vi "new.vi"() -> ()   [LabVIEW 2019]
uses:
  <vilib>/Instr/_visa.llb/VISA Configure Serial Port (Instr).vi
panel:
  out "3.3V REG":cluster{dbl, dbl}(graph)
  out "3.3 current":dbl caption="Current Temperature\n(Celsius)"
  out "3.3V voltage":dbl caption="Current Temperature\n(Celsius)"
  out "5V REG":cluster{dbl, dbl}(graph)
  out "5V current":dbl caption="Current Temperature\n(Celsius)"
  out "Currents":cluster{dbl, dbl}(graph)
  in  "project name":string
  out "Bus Voltage":dbl(graph)
  out "5V voltage":dbl caption="Current Temperature\n(Celsius)"
  in  "StartConverter":bool
  out "String":string
  in  "VISA resource name":refnum<visa-resource-name>="COM4"
  out "LOAD current":dbl caption="Current Temperature\n(Celsius)"
  out "PVA current":dbl caption="Current Temperature\n(Celsius)"
  out "BUS voltage":dbl caption="Current Temperature\n(Celsius)"
  out "Still in Sync":bool
  in  "stop":bool
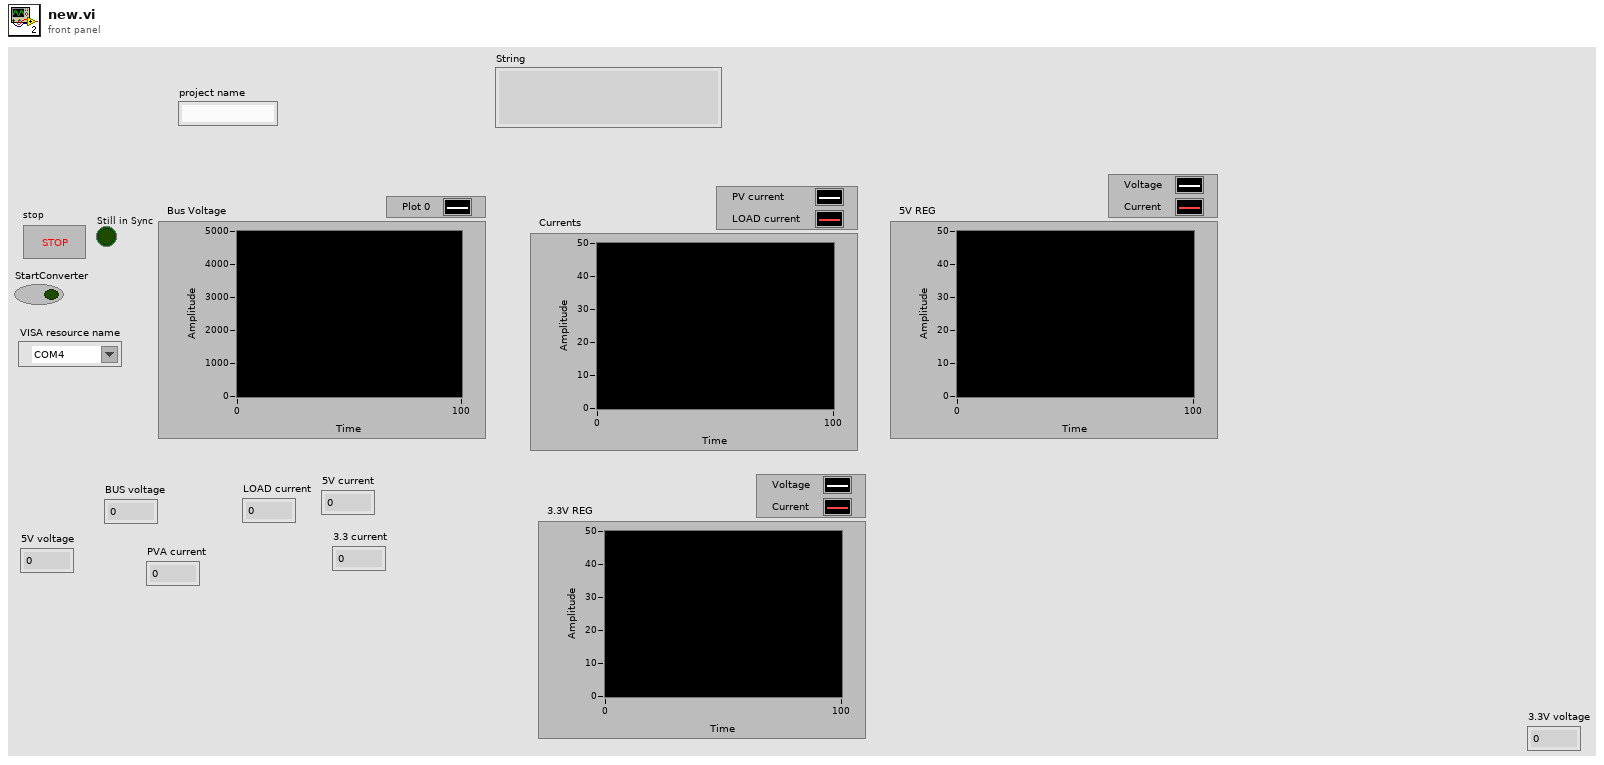
[diagram p1: front panel]
types:
  T1 = cluster{u16, u16, u16, u16, u16, u16, u16, u16, u16}
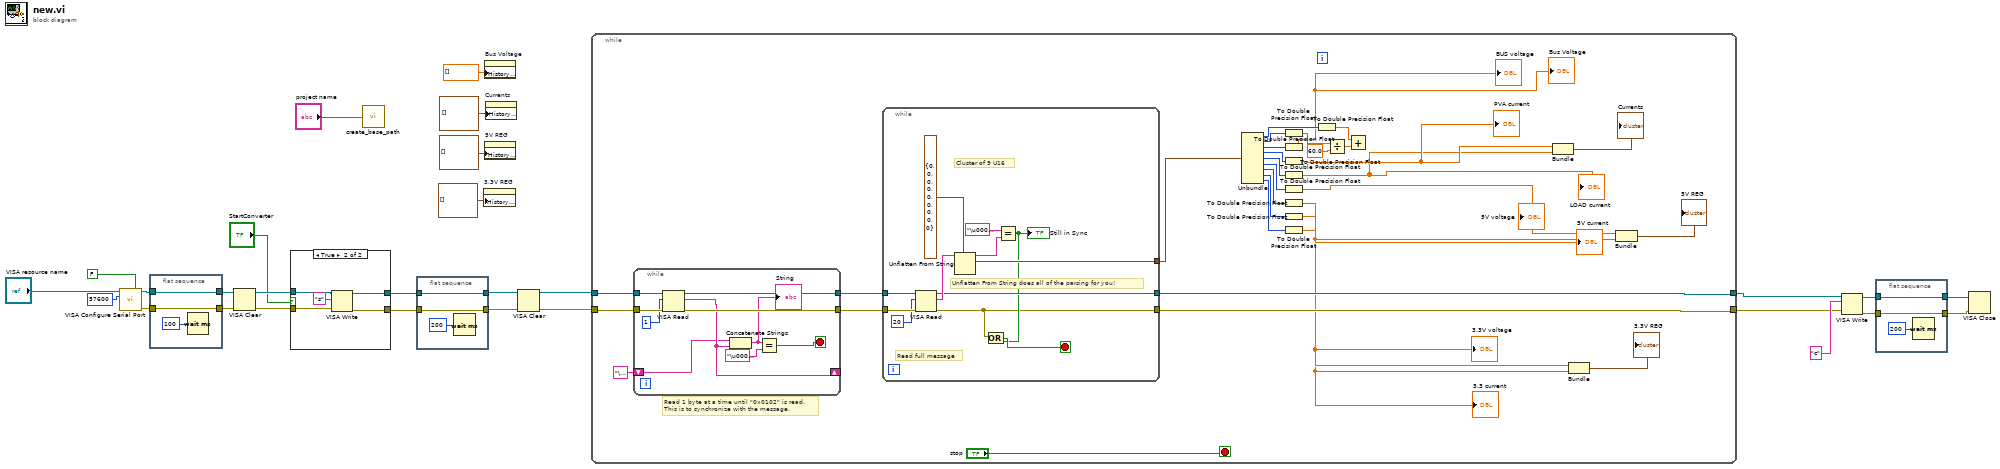
[diagram p0: block diagram]
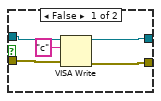
[diagram p2: hidden frame]
diagram:
  n1 = call-poly "VISA Configure Serial Port"("VISA resource name"="VISA resource name", "Enable Termination\nChar (T)"=FALSE ("Enable Termination\nChar (T)"), "baud rate (9600)"=u32 57600) -> ("VISA resource name out"=w25:refnum<visa-resource-name>, "error out"=w24:errorcluster)  [unwired: 11 in]
  n2 = flat-sequence {
    tunnel: w24 -> [w30]
    tunnel: [w30] -> w23
    tunnel: [w29] -> w22
    tunnel: w25 -> [w29]
    frame #0 {
      n3 = Wait (ms)(milliseconds to wait=u32 100) -> ()  [unwired: 1 out]
    }
  }
  n4 = VISA Clear(VISA resource name=w22, error in (no error)=w23) -> (VISA resource name out=w21:refnum<visa-resource-name>, error out=w20:errorcluster)
  n5 = case shown="True" "StartConverter" {
    tunnel: w21 -> [w35 w41]
    tunnel: [w33 w40] -> w18
    tunnel: w20 -> [w34 w39]
    tunnel: [w32 w38] -> w17
    frame False {
      n6 = VISA Write(VISA resource name=w35, write buffer="c", error in (no error)=w34) -> (VISA resource name out=w33:refnum<visa-resource-name>, error out=w32:errorcluster)  [unwired: 1 out]
    }
    frame True {
      n7 = VISA Write(VISA resource name=w41, write buffer="s", error in (no error)=w39) -> (VISA resource name out=w40:refnum<visa-resource-name>, error out=w38:errorcluster)  [unwired: 1 out]
    }
  }
  n8 = call "create_base_path.vi"("project name"="project name") -> ()  [unwired: 1 out]
  n9 = flat-sequence {
    tunnel: w17 -> [w43]
    tunnel: [w43] -> w14
    tunnel: [w42] -> w16
    tunnel: w18 -> [w42]
    frame #0 {
      n10 = Wait (ms)(milliseconds to wait=u32 200) -> ()  [unwired: 1 out]
    }
  }
  n11 = property on="3.3V REG" class="WFChart (strict)"("History Data"=cluster{dbl, dbl}[] []) -> ()  [unwired: 2 in, 2 out]
  n12 = property on="Bus Voltage" class="WFChart (strict)"("History Data"=dbl[] []) -> ()  [unwired: 2 in, 2 out]
  n13 = property on="5V REG" class="WFChart (strict)"("History Data"=cluster{dbl, dbl}[] []) -> ()  [unwired: 2 in, 2 out]
  n14 = property on="Currents" class="WFChart (strict)"("History Data"=cluster{dbl, dbl}[] []) -> ()  [unwired: 2 in, 2 out]
  n15 = VISA Clear(VISA resource name=w16, error in (no error)=w14) -> (VISA resource name out=w15:refnum<visa-resource-name>, error out=w13:errorcluster)
  n16 = while {
    tunnel: w13 -> [w74]
    tunnel: [w60] -> w10
    tunnel: [w61] -> w11
    tunnel: w15 -> [w62]
    stop <- "stop" stop-if-true
    # "Read 1 byte at a time until \"0x0102\" is read.\nThis is to synchronize with the message."
    n17 = while {
      tunnel: w62 -> [w96]
      tunnel: w74 -> [w98]
      tunnel: [w97] -> w75
      tunnel: [w93] -> w76
      shift-right: [w90] -> _
      shift-left: "\u0000" ("read buffer") -> [w89]
      stop <- w91 stop-if-true
      n18 = VISA Read(VISA resource name=w96, byte count=u32 1, error in (no error)=w98) -> (VISA resource name out=w93:refnum<visa-resource-name>, read buffer=w90:string, error out=w97:errorcluster)  [unwired: 1 out]
      n19 = Concatenate Strings(w89, w90) -> (w92:string)
      "String" <- w92
      n20 = Equal?(x=w92, y="\u0001\u0002") -> (x = y?=w91:bool)
    }
    n21 = while {
      tunnel: w75 -> [w88]
      tunnel: w76 -> [w87]
      tunnel: [w77] -> w60
      tunnel: [w81] -> w61
      tunnel: [w79] -> w72
      stop <- w80 stop-if-true
      # "Unflatten From String does all of the parsing for you!"
      # "Cluster of 9 U16"
      # "Read full message"
      n22 = VISA Read(VISA resource name=w87, byte count=u32 20, error in (no error)=w88) -> (VISA resource name out=w81:refnum<visa-resource-name>, read buffer=w85:string, error out=w77:errorcluster)  [unwired: 1 out]
      n23 = Unflatten From String(type=T1 {0, 0, 0, 0, 0, 0, 0, 0, 0}, binary string=w85) -> (rest of the binary string=w83:string, value=w79:T1)  [unwired: 3 in, 1 out]
      n24 = Equal?(x="\u0002\u0001", y=w83) -> (x = y?=w78:bool)
      "Still in Sync" <- w78
      n25 = Or(x=w77, y=w78) -> (x .or. y?=w80:bool)
    }
    n26 = Unbundle(w72) -> (w71:u16, w70:u16, w65:u16, w64:u16, w63:u16, w58:u16, w53:u16, w52:u16, w51:u16)
    n27 = To Double Precision Float(number=w70) -> (double precision float=w68:dbl)
    n28 = To Double Precision Float(number=w65) -> (double precision float=→"BUS voltage" →"Bus Voltage":dbl)
    n29 = To Double Precision Float(number=w64) -> (double precision float=w56:dbl)
    "PVA current" <- w56
    n30 = To Double Precision Float(number=w63) -> (double precision float=w55:dbl)
    "LOAD current" <- w55
    n31 = To Double Precision Float(number=w58) -> (double precision float=w49:dbl)
    "5V voltage" <- w49
    n32 = To Double Precision Float(number=w53) -> (double precision float=w48:dbl)
    "5V current" <- w48
    n33 = To Double Precision Float(number=w52) -> (double precision float=w46:dbl)
    "3.3V voltage" <- w46
    n34 = To Double Precision Float(number=w51) -> (double precision float=w45:dbl)
    "3.3 current" <- w45
    n35 = To Double Precision Float(number=w71) -> (double precision float=w67:dbl)
    n36 = Divide(x=w68, y=60.0) -> (x/y=w66:dbl)
    n37 = Add(x=w67, y=w66) -> ()  [unwired: 1 out]
    n38 = Bundle(w56, w55) -> (→"Currents":cluster{dbl, dbl})  [unwired: 1 in]
    n39 = Bundle(w46, w45) -> (→"3.3V REG":cluster{dbl, dbl})  [unwired: 1 in]
    n40 = Bundle(w49, w48) -> (→"5V REG":cluster{dbl, dbl})  [unwired: 1 in]
  }
  n41 = VISA Write(VISA resource name=w11, write buffer="c", error in (no error)=w10) -> (VISA resource name out=w9:refnum<visa-resource-name>, error out=w8:errorcluster)  [unwired: 1 out]
  n42 = flat-sequence {
    tunnel: w8 -> [w100]
    tunnel: [w100] -> w7
    tunnel: [w99] -> w6
    tunnel: w9 -> [w99]
    frame #0 {
      n43 = Wait (ms)(milliseconds to wait=u32 200) -> ()  [unwired: 1 out]
    }
  }
  n44 = VISA Close(VISA resource name=w6, error in (no error)=w7) -> ()  [unwired: 1 out]
